vi "Spacer Position.vi"() -> ()   [LabVIEW 2020]
doc: "Este programa executa calculos para determinar o número de espaçadores e a sua respectiva posição."
uses:
  controles/SP dados de entrada.ctl
  controles/SP data.ctl
panel:
  out "Etapa":string="Término do programa"
  in  "Próximo":bool
  in  "Parar 2":bool
  out "Dados":enum32{"Dados", "Análise"}(tab)
  in  "Condutor":T1={"Pc (N/m)"=18.35, "Mod.Young (GPa)"=65.0, "Dil.Term.c (u/°C)"=20.9, "Seção trans. (mm²)"=496.0, "Tração EDS (N)"=18350.0, "Tração Lim.orig (N)"=0.0, "Tração Text (N)"=0.0} {"Tração Text (N)" min=0.0 max=1000000.0 step=0.01 format="%.2f"; "Tração Lim.orig (N)" min=0.0 max=1000000.0 step=0.01 format="%.2f"; "Pc (N/m)" min=1.0 max=100.0 step=0.01 format="%#.2g"; "Mod.Young (GPa)" min=1.0 max=500.0 step=0.001 format="%#.3f"; "Dil.Term.c (u/°C)" min=0.0 max=40.0 step=0.001 format="%#.2f"; "Seção trans. (mm²)" min=0.0 max=2000.0 step=0.001 format="%#.6f"; "Tração EDS (N)" min=1000.0 max=200000.0 step=0.01 format="%.2f"}
  in  "Suporte":T2={"Ps (N/m)"=10.0, "Mod.Young (GPa)"=112.0, "Dil.Term.c (u/°C)"=1.6, "Seção trans. (mm²)"=396.0, "Tração EDS (N)"=13250.0, "AT sup (N)"=0.0, "Flecha sup AT (m)"=0.0} {"AT sup (N)" min=0.0 max=2000.0 step=0.001 format="%#.6f"; "Tração EDS (N)" min=0.0 max=500000.0 step=0.01 format="%#.6f"; "Ps (N/m)" min=1.0 max=200.0 step=0.01; "Mod.Young (GPa)" min=1.0 max=500.0 step=0.001 format="%#.3f"; "Dil.Term.c (u/°C)" min=0.0 max=40.0 step=0.001 format="%#_3f"; "Seção trans. (mm²)" min=0.0 max=2000.0 step=0.001 format="%#.6f"}
  in  "Projeto":T3={"Temp. EDS (°C)"=25.0, "Limite orig (°C)"=60.0, "Limite est (°C)"=100.0, "N° Cabo/Fase"=4} {"N° Cabo/Fase" min=1 max=8 step=1; "Limite est (°C)" min=-50.0 max=300.0 step=0.01; "Temp. EDS (°C)" min=-50.0 max=100.0 step=0.01; "Limite orig (°C)" min=0.0 max=300.0 step=0.01}
  in  "Vão":T4={"Extensão. (m)"=700.0, "Desnível (m)"=20.0, "Ext lim subvão (m)"=20.0, "Flecha 60 (°C)"=0.0} {"Ext lim subvão (m)" min=0.0 max=500.0 step=0.01; "Flecha 60 (°C)" min=0.0 max=500.0 step=0.01; "Extensão. (m)" min=100.0 max=2000.0 step=0.01; "Desnível (m)" min=0.0 max=500.0 step=0.01}
  in  "Subaba de dados":enum32{"Espaçadores", "Subvão", "Cabo Suporte"}(tab)
  out "N Espaçadores":dbl=8.0
  out "Posição no vão (m)":dbl[](array[numeric])
  out "Tração cond. (N)":dbl=17448.399999999863
  out "Extensão c/ 55% (m)":dbl
  out "Flecha lim.calc (m)":dbl
  out "Comp Calc (m)":dbl=17448.399999999863
  out "Tração EDS (N)":dbl=83817.19488812913
  out "Tração Test (N)":dbl=83817.19488812913
  out "Flecha Test (m)":dbl
  out "Gráfico":cluster{dbl[], dbl[]}[](graph)
  in  "Gravar":bool
  # "Preenchimento de dados"
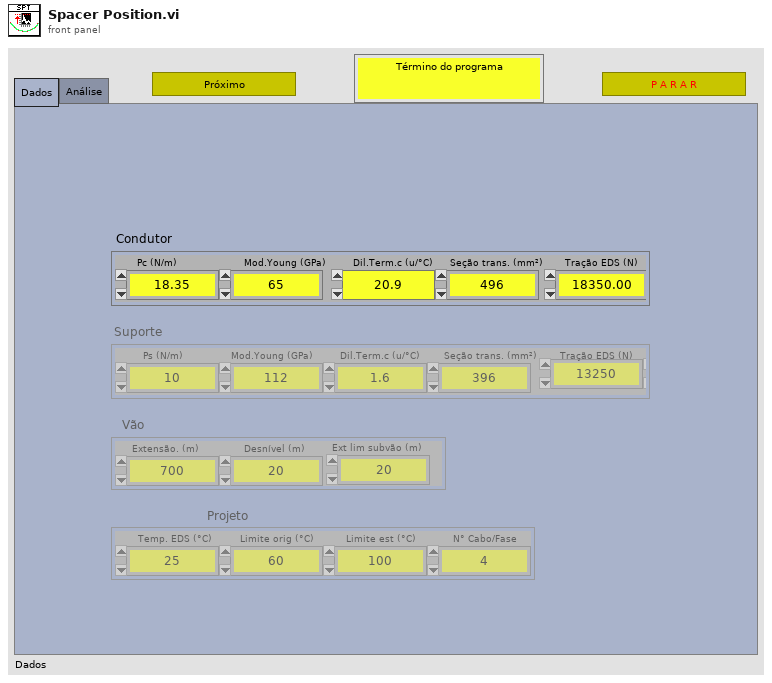
[diagram p1: front panel]
types:
  T1 = cluster{"Pc (N/m)":dbl, "Mod.Young (GPa)":dbl, "Dil.Term.c (u/°C)":dbl, "Seção trans. (mm²)":dbl, "Tração EDS (N)":dbl, "Tração Lim.orig (N)":dbl, "Tração Text (N)":dbl}
  T2 = cluster{"Ps (N/m)":dbl, "Mod.Young (GPa)":dbl, "Dil.Term.c (u/°C)":dbl, "Seção trans. (mm²)":dbl, "Tração EDS (N)":dbl, "AT sup (N)":dbl, "Flecha sup AT (m)":dbl}
  T3 = cluster{"Temp. EDS (°C)":dbl, "Limite orig (°C)":dbl, "Limite est (°C)":dbl, "N° Cabo/Fase":u32}
  T4 = cluster{"Extensão. (m)":dbl, "Desnível (m)":dbl, "Ext lim subvão (m)":dbl, "Flecha 60 (°C)":dbl}
  T5 = typedef "SP data.ctl" = cluster{"Condutor":cluster{"Pc (N/m)":dbl, "Mod.Young (N/m²)":dbl, "Dil.Term.c (m/°C)":dbl, "Área  (m²)":dbl, "Tração EDS (N)":dbl, "Tração Torig(N)":dbl, "Tração Talta (N)":dbl}, "Suporte":cluster{"Ps (N/m)":dbl, "Es (N/m²)":dbl, "DTc (1/°C)":dbl, "Área sup (m²)":dbl, "Tração EDS sup (N)":dbl, "Tração AT sup (N)":dbl, "Flecha sup AT (m)":dbl}, "Projeto":cluster{"Temp. EDS (°C)":dbl, "Lim.original (°C)":dbl, "Lim.extend. (°C)":dbl, "N. cabo/fase":dbl}, "Vetor de dados":cluster{"Coor.X.esp":dbl[], "Coor.Y.Esp.":dbl[], "Sub.vao X":dbl[], "Sub.vao Y":dbl[], "CoordY.sup":dbl[], "CoordX.sup":dbl[]}, "Subvão":cluster{"N. Esp.":dbl, "F.lim (m)":dbl, "Ext.calc":dbl, "Ext.definido":dbl, "Comp.cabo":dbl, "Ext.55%":dbl, "Tração sub\nAT (N)":dbl, "Ext.sel.":dbl, "Flecha lim.\ncalc (m)":dbl}, "Vão":cluster{"Extensão (m)":dbl, "Desnivel (m)":dbl, "Ext.Lim sub (m)":dbl, "Flecha à 60 °C":dbl}}
  T6 = typedef "SP dados de entrada.ctl" = enum16{"Iniciar", "Aguardar", "Condutor", "Suporte", "Vão", "Projeto", "Atualizar UI", "Mensagem", "Calcular", "Análise dos dados", "Fim"}
  T7 = enum8{"Enabled", "Disabled", "Disabled and Grayed Out"}
  T8 = cluster{"CoordX.sup":dbl[], "CoordY.sup":dbl[]}[]
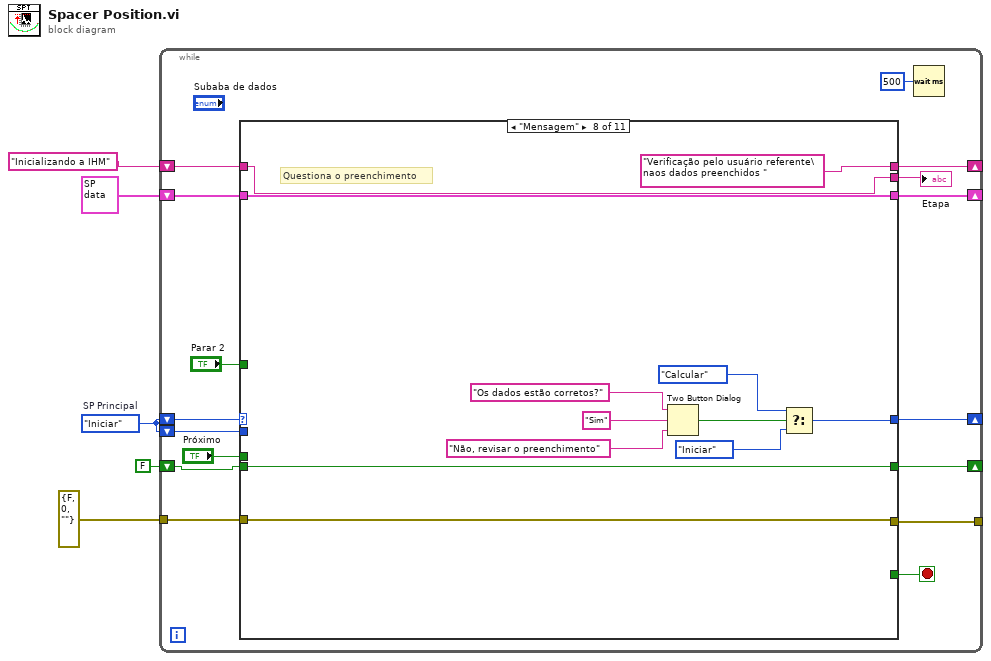
[diagram p0: block diagram]
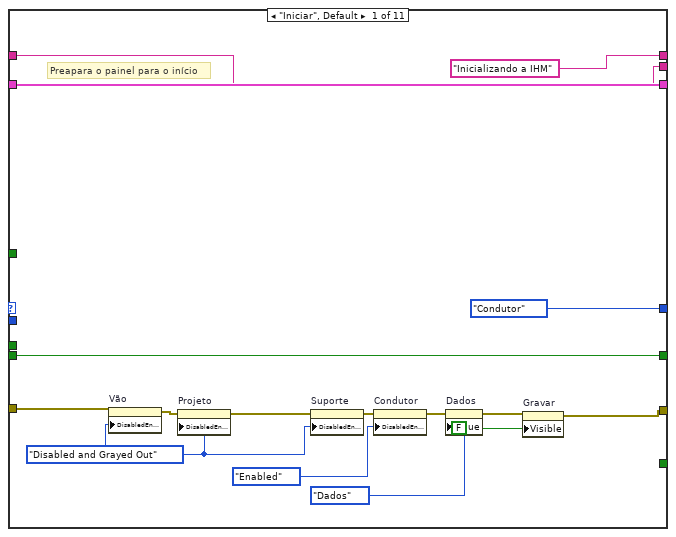
[diagram p2: hidden frame]
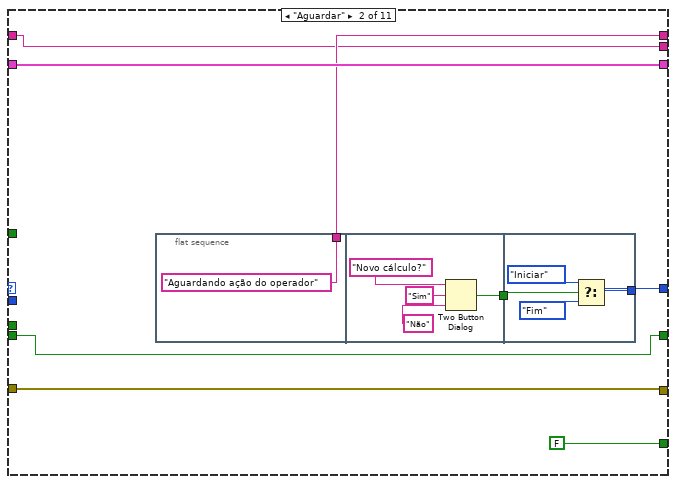
[diagram p3: hidden frame]
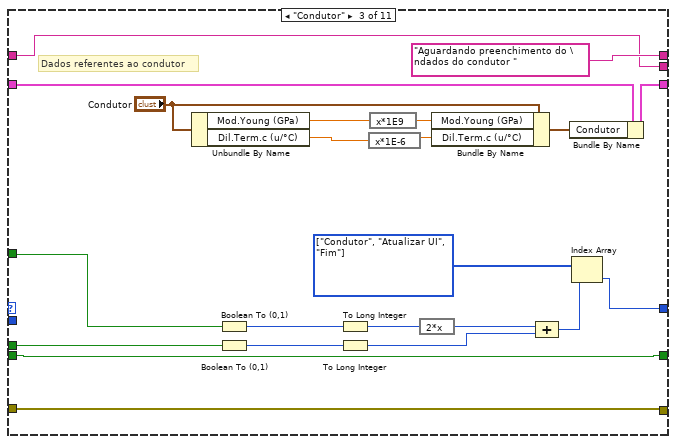
[diagram p4: hidden frame]
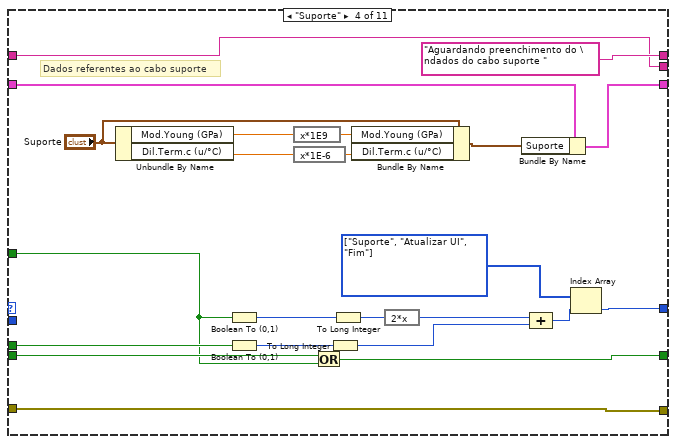
[diagram p5: hidden frame]
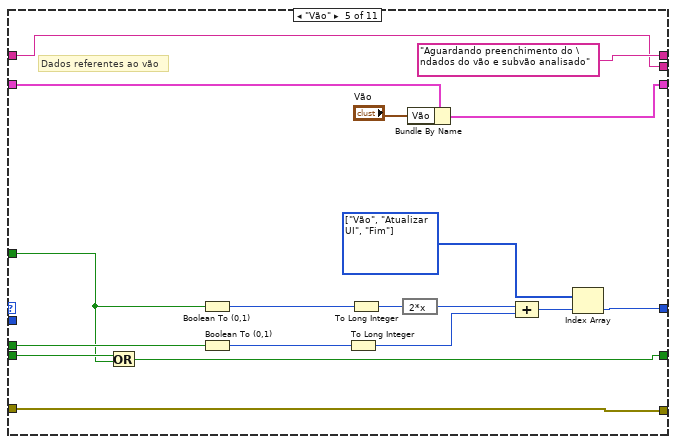
[diagram p6: hidden frame]
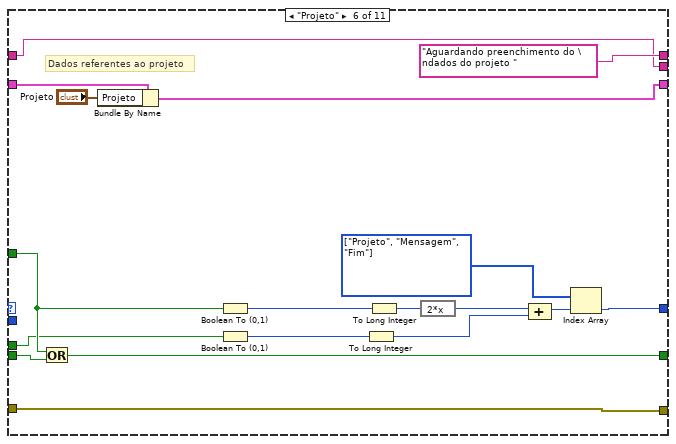
[diagram p7: hidden frame]
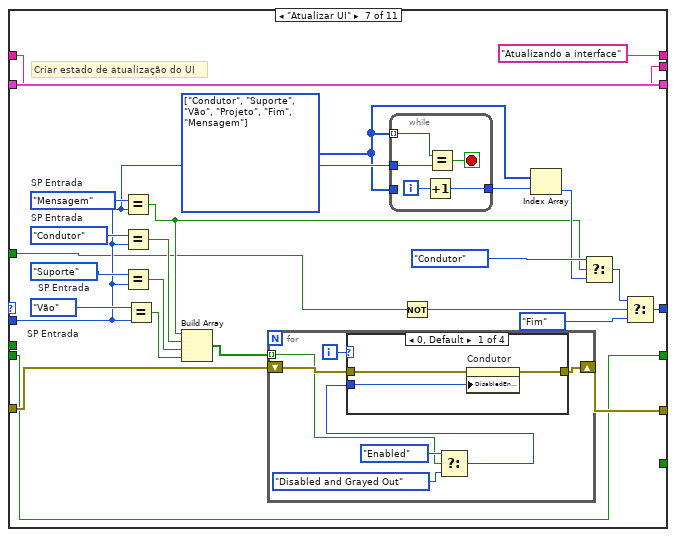
[diagram p8: hidden frame]
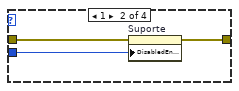
[diagram p9: hidden frame]
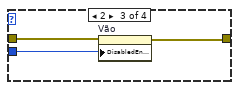
[diagram p10: hidden frame]
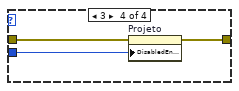
[diagram p11: hidden frame]
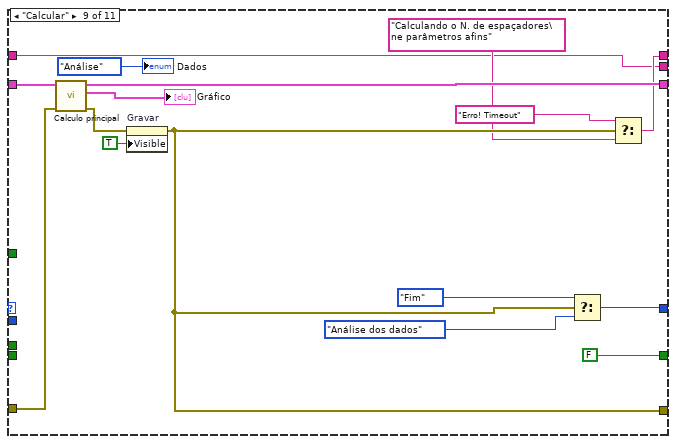
[diagram p12: hidden frame]
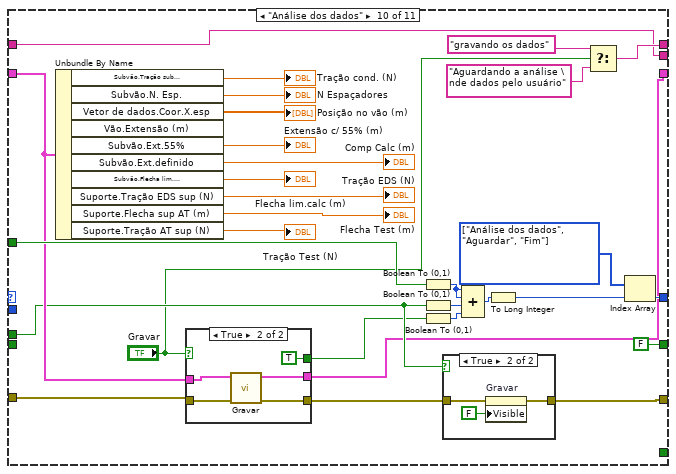
[diagram p13: hidden frame]
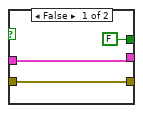
[diagram p14: hidden frame]
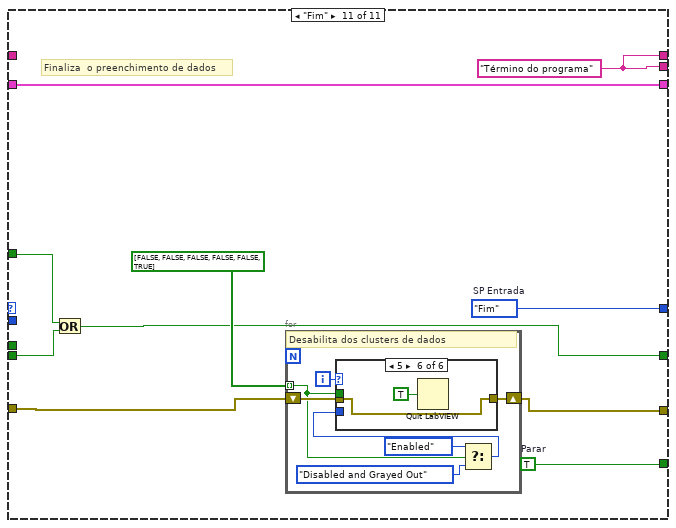
[diagram p16: hidden frame]
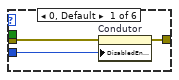
[diagram p17: hidden frame]
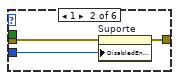
[diagram p18: hidden frame]
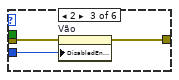
[diagram p19: hidden frame]
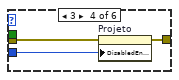
[diagram p20: hidden frame]
diagram:
  w3 = SP_dados_de_entrada."Iniciar"  # SP Principal
  n1 = while {
    shift-right: [w20] -> _
    shift-left: w3 -> [w21]
    shift-right: [w17] -> _
    shift-left: T5 {"Condutor"={"Pc (N/m)"=0.0, "Mod.Young (N/m²)"=0.0, "Dil.Term.c (m/°C)"=0.0, "Área  (m²)"=0.0, "Tração EDS (N)"=0.0, "Tração Torig(N)"=0.0, "Tração Talta (N)"=0.0}, "Suporte"={"Ps (N/m)"=0.0, "Es (N/m²)"=0.0, "DTc (1/°C)"=0.0, "Área sup (m²)"=0.0, "Tração EDS sup (N)"=0.0, "Tração AT sup (N)"=0.0, "Flecha sup AT (m)"=0.0}, "Projeto"={"Temp. EDS (°C)"=0.0, "Lim.original (°C)"=0.0, "Lim.extend. (°C)"=0.0, "N. cabo/fase"=1.0}, "Vetor de dados"={"Coor.X.esp"=[], "Coor.Y.Esp."=[], "Sub.vao X"=[], "Sub.vao Y"=[], "CoordY.sup"=[], "CoordX.sup"=[]}, "Subvão"={"N. Esp."=0.0, "F.lim (m)"=0.0, "Ext.calc"=0.0, "Ext.definido"=0.0, "Comp.cabo"=0.0, "Ext.55%"=0.0, "Tração sub\nAT (N)"=0.0, "Ext.sel."=0.0, "Flecha lim.\ncalc (m)"=0.0}, "Vão"={"Extensão (m)"=0.0, "Desnivel (m)"=0.0, "Ext.Lim sub (m)"=0.0, "Flecha à 60 °C"=0.0}} ("SP Dados In") -> [w18]
    shift-left: w3 -> [w15]
    tunnel: errorcluster {"status"=FALSE, "code"=0, "source"=""} ("error in") -> [w14]
    tunnel: [w9] -> _
    shift-right: [w12] -> _
    shift-left: FALSE ("T button?") -> [w11]
    shift-right: [w8] -> _
    shift-left: "Inicializando a IHM" ("Etapa") -> [w6]
    stop <- w19 stop-if-true
    n2 = case shown="\"Mensagem\"" w21 {
      tunnel: [SP_dados_de_entrada."Condutor" ("SP Entrada") w39 w73 w98 w116 w134 w149 w192 w201 w230 w264] -> w20
      tunnel: [_ FALSE ("Parar") _ _ _ _ _ _ _ _ w263] -> w19
      tunnel: [w37 w45 w74 w77 w114 w119 w157 w186 w207 w221 w262] -> w17
      tunnel: w18 -> [w37 w45 w75 w79 w115 w133 w157 w186 w211 w225 w262]
      tunnel: w15 -> [_ _ _ _ _ _ w142 _ _ _ _]
      tunnel: w14 -> [w23 w43 w72 w97 w113 w131 w153 w195 w210 w226 w261]
      tunnel: [w28 w43 w72 w97 w113 w131 w152 w195 w206 w222 w260] -> w9
      tunnel: "Próximo" -> [_ _ w70 w95 w103 w120 _ _ _ w224 _]
      tunnel: [w33 w44 w69 w93 w111 w130 w140 w188 FALSE ("T button?") FALSE ("T button?") w258] -> w12
      tunnel: w11 -> [w33 w44 w69 w94 w112 w122 w140 w188 _ _ w257]
      tunnel: "Parar 2" -> [_ _ w63 w88 w102 w121 w139 _ _ w228 w256]
      tunnel: ["Inicializando a IHM" ("Etapa") w41 "Aguardando preenchimento do \ndados do condutor " ("Etapa") "Aguardando preenchimento do \ndados do cabo suporte " ("Etapa") "Aguardando preenchimento do \ndados do vão e subvão analisado" ("Etapa") "Aguardando preenchimento do \ndados do projeto " ("Etapa") "Atualizando a interface" ("Etapa") "Verificação pelo usuário referente\naos dados preenchidos " ("Etapa") w199 w217 w255] -> w8
      tunnel: [w25 w38 w61 w85 w101 w118 w136 w185 w197 w213 w255] -> w7
      tunnel: w6 -> [w25 w38 w61 w85 w101 w118 w136 w185 w197 w213 _]
      frame "Iniciar", Default {
        w22 = T7."Disabled and Grayed Out" ("Disabled")
        # "Preapara o painel para o início"
        n3 = property on="Vão" class="Clust (strict)"(error in=w23, "DisabledEnum"=w22) -> (error out=w24:errorcluster)  [unwired: 1 in, 1 out]
        n4 = property on="Projeto" class="Clust (strict)"(error in=w24, "DisabledEnum"=w22) -> (error out=w36:errorcluster)  [unwired: 1 in, 1 out]
        n5 = property on="Suporte" class="Clust (strict)"(error in=w36, "DisabledEnum"=w22) -> (error out=w35:errorcluster)  [unwired: 1 in, 1 out]
        n6 = property on="Condutor" class="Clust (strict)"(error in=w35, "DisabledEnum"=T7."Enabled" ("Disabled")) -> (error out=w32:errorcluster)  [unwired: 1 in, 1 out]
        n7 = property on="Dados" class="TabCtl (strict)"(error in=w32, "Value"=enum32{"Dados", "Análise"}."Dados" ("Dados")) -> (error out=w29:errorcluster)  [unwired: 1 in, 1 out]
        n8 = property on="Gravar" class="Bool"(error in=w29, "Visible"=FALSE) -> (error out=w28:errorcluster)  [unwired: 1 in, 1 out]
      }
      frame "Aguardar" {
        n9 = flat-sequence {
          tunnel: ["Aguardando ação do operador" ("Etapa")] -> w41
          tunnel: [w47] -> w40
          tunnel: w40 -> [w53]
          tunnel: [w51] -> w39
          frame #0 {
          }
          frame #1 {
            n10 = Two Button Dialog(message="Novo cálculo?" ("T button name (\"OK\")"), 1:"Não" ("F button name (\"Cancel\")"), 2:"Sim" ("message")) -> (T button?=w47:bool)
          }
          frame #2 {
            n11 = Select(t=SP_dados_de_entrada."Iniciar" ("SP Entrada"), s=w53, f=SP_dados_de_entrada."Fim" ("SP Entrada")) -> (s? t:f=w51:T6)
          }
        }
      }
      frame "Condutor" {
        w76 = T6[] [enum."Condutor", enum."Atualizar UI", enum."Fim"] items=["Iniciar", "Aguardar", "Condutor", "Suporte", "Vão", "Projeto", "Atualizar UI", "Mensagem", "Calcular", "Análise dos dados", "Fim"]
        # "Dados referentes ao condutor"
        n12 = Unbundle By Name("Condutor") -> ("Mod.Young (GPa)"=w59:dbl, "Dil.Term.c (u/°C)"=w56:dbl)
        n13 = Boolean To (0,1)(Boolean=w63) -> (0, 1=w65:i16)
        n14 = Boolean To (0,1)(Boolean=w70) -> (0, 1=w71:i16)
        n15 = To Long Integer(number=w65) -> (32bit integer=w64:i32)
        n16 = To Long Integer(number=w71) -> (32bit integer=w67:i32)
        n17 = expression code="x*1E-6"(w56) -> (w55:dbl)
        n18 = expression code="x*1E9"(w59) -> (w58:dbl)
        n19 = expression code="2*x"(w64) -> (w62:i32)
        n20 = Bundle By Name(cluster="Condutor", "Mod.Young (GPa)"=w58, "Dil.Term.c (u/°C)"=w55) -> (w57:T1)
        n21 = Compound Arithmetic op=ADD(w62, w67) -> (w66:i32)
        n22 = Bundle By Name(cluster=w75, "Condutor"=w57) -> (w74:T5)
        n23 = Index Array(array=w76, index=w66) -> (element=w73:T6)
      }
      frame "Suporte" {
        w99 = T6[] [enum."Suporte", enum."Atualizar UI", enum."Fim"] items=["Iniciar", "Aguardar", "Condutor", "Suporte", "Vão", "Projeto", "Atualizar UI", "Mensagem", "Calcular", "Análise dos dados", "Fim"]
        # "Dados referentes ao cabo suporte"
        n24 = Unbundle By Name("Suporte") -> ("Mod.Young (GPa)"=w84:dbl, "Dil.Term.c (u/°C)"=w82:dbl)
        n25 = Boolean To (0,1)(Boolean=w88) -> (0, 1=w91:i16)
        n26 = Boolean To (0,1)(Boolean=w95) -> (0, 1=w96:i16)
        n27 = expression code="x*1E9"(w84) -> (w83:dbl)
        n28 = expression code="x*1E-6"(w82) -> (w81:dbl)
        n29 = Or(x=w94, y=w88) -> (x .or. y?=w93:bool)
        n30 = To Long Integer(number=w96) -> (32bit integer=w87:i32)
        n31 = To Long Integer(number=w91) -> (32bit integer=w90:i32)
        n32 = Bundle By Name(cluster="Suporte", "Mod.Young (GPa)"=w83, "Dil.Term.c (u/°C)"=w81) -> (w78:T2)
        n33 = expression code="2*x"(w90) -> (w89:i32)
        n34 = Bundle By Name(cluster=w79, "Suporte"=w78) -> (w77:T5)
        n35 = Compound Arithmetic op=ADD(w89, w87) -> (w86:i32)
        n36 = Index Array(array=w99, index=w86) -> (element=w98:T6)
      }
      frame "Vão" {
        w117 = T6[] [enum."Vão", enum."Atualizar UI", enum."Fim"] items=["Iniciar", "Aguardar", "Condutor", "Suporte", "Vão", "Projeto", "Atualizar UI", "Mensagem", "Calcular", "Análise dos dados", "Fim"]
        # "Dados referentes ao vão"
        n37 = Or(x=w112, y=w102) -> (x .or. y?=w111:bool)
        n38 = Boolean To (0,1)(Boolean=w102) -> (0, 1=w108:i16)
        n39 = Boolean To (0,1)(Boolean=w103) -> (0, 1=w109:i16)
        n40 = To Long Integer(number=w109) -> (32bit integer=w105:i32)
        n41 = To Long Integer(number=w108) -> (32bit integer=w107:i32)
        n42 = expression code="2*x"(w107) -> (w106:i32)
        n43 = Bundle By Name(cluster=w115, "Vão"="Vão") -> (w114:T5)
        n44 = Compound Arithmetic op=ADD(w106, w105) -> (w104:i32)
        n45 = Index Array(array=w117, index=w104) -> (element=w116:T6)
      }
      frame "Projeto" {
        w135 = T6[] [enum."Projeto", enum."Mensagem", enum."Fim"] items=["Iniciar", "Aguardar", "Condutor", "Suporte", "Vão", "Projeto", "Atualizar UI", "Mensagem", "Calcular", "Análise dos dados", "Fim"]
        # "Dados referentes ao projeto"
        n46 = Or(x=w121, y=w122) -> (x .or. y?=w130:bool)
        n47 = Bundle By Name(cluster=w133, "Projeto"="Projeto") -> (w119:T5)
        n48 = Boolean To (0,1)(Boolean=w121) -> (0, 1=w127:i16)
        n49 = Boolean To (0,1)(Boolean=w120) -> (0, 1=w128:i16)
        n50 = To Long Integer(number=w128) -> (32bit integer=w124:i32)
        n51 = To Long Integer(number=w127) -> (32bit integer=w126:i32)
        n52 = expression code="2*x"(w126) -> (w125:i32)
        n53 = Compound Arithmetic op=ADD(w125, w124) -> (w123:i32)
        n54 = Index Array(array=w135, index=w123) -> (element=w134:T6)
      }
      frame "Atualizar UI" {
        w147 = SP_dados_de_entrada."Mensagem"  # SP Entrada
        w138 = T6[] [enum."Condutor", enum."Suporte", enum."Vão", enum."Projeto", enum."Fim", enum."Mensagem"] items=["Iniciar", "Aguardar", "Condutor", "Suporte", "Vão", "Projeto", "Atualizar UI", "Mensagem", "Calcular", "Análise dos dados", "Fim"]
        w158 = SP_dados_de_entrada."Vão"  # SP Entrada
        w159 = SP_dados_de_entrada."Suporte"  # SP Entrada
        w160 = SP_dados_de_entrada."Condutor"  # SP Entrada
        # "Criar estado de atualização do UI"
        n55 = Equal?(x=w147, y=w142) -> (x = y?=w141:bool)
        n56 = Equal?(x=w160, y=w142) -> (x = y?=w156:bool)
        n57 = Equal?(x=w159, y=w142) -> (x = y?=w155:bool)
        n58 = Equal?(x=w158, y=w142) -> (x = y?=w148:bool)
        n59 = Build Array(w141, w156, w155, w148) -> (w154:bool[])
        n60 = for {
          shift-right: [w166] -> w152
          shift-left: w153 -> [w165]
          tunnel: w154 -> [w161] mode=indexing
          i -> [w167]
          n61 = Select(t=T7."Enabled" ("Disabled"), s=w161, f=T7."Disabled and Grayed Out" ("Disabled")) -> (s? t:f=w162:T7)
          n62 = case shown="0, Default" w167 {
            tunnel: [w170 w173 w175 w179] -> w166
            tunnel: w165 -> [w168 w172 w174 w178]
            tunnel: w162 -> [w169 w171 w176 w177]
            frame 0, Default {
              n63 = property on="Condutor" class="Clust (strict)"(error in=w168, "DisabledEnum"=w169) -> (error out=w170:errorcluster)  [unwired: 1 in, 1 out]
            }
            frame 1 {
              n64 = property on="Suporte" class="Clust (strict)"(error in=w172, "DisabledEnum"=w171) -> (error out=w173:errorcluster)  [unwired: 1 in, 1 out]
            }
            frame 2 {
              n65 = property on="Vão" class="Clust (strict)"(error in=w174, "DisabledEnum"=w176) -> (error out=w175:errorcluster)  [unwired: 1 in, 1 out]
            }
            frame 3 {
              n66 = property on="Projeto" class="Clust (strict)"(error in=w178, "DisabledEnum"=w177) -> (error out=w179:errorcluster)  [unwired: 1 in, 1 out]
            }
          }
        }
        n67 = while {
          tunnel: w138 -> [w180] mode=indexing
          tunnel: w138 -> [_]
          tunnel: [w182] -> w146
          tunnel: w142 -> [w181]
          i -> [w183]
          stop <- w184 stop-if-true
          n68 = Increment(x=w183) -> (x+1=w182:i32)
          n69 = Equal?(x=w180, y=w181) -> (x = y?=w184:bool)
        }
        n70 = Not(x=w139) -> (.not. x?=w151:bool)
        n71 = Index Array(array=w138, index=w146) -> (element=w144:T6)
        n72 = Select(t=SP_dados_de_entrada."Condutor" ("f"), s=w141, f=w144) -> (s? t:f=w143:T6)
        n73 = Select(t=w143, s=w151, f=SP_dados_de_entrada."Fim") -> (s? t:f=w149:T6)
      }
      frame "Mensagem" {
        # "Questiona o preenchimento"
        n74 = Two Button Dialog(message="Os dados estão corretos?" ("T button name (\"OK\")"), 1:"Não, revisar o preenchimento" ("F button name (\"Cancel\")"), 2:"Sim" ("message")) -> (T button?=w189:bool)
        n75 = Select(t=SP_dados_de_entrada."Calcular" ("SP Entrada"), s=w189, f=SP_dados_de_entrada."Iniciar" ("SP Entrada")) -> (s? t:f=w192:T6)
      }
      frame "Calcular" {
        n76 = call "Calculo principal.vi"("error in"=w210, "Dados SP"=w211) -> ("error out"=w208:errorcluster, "Gráfico"=→"Gráfico":T8, "Dados SP Out"=w207:T5)  [unwired: 7 in]
        n77 = property on="Gravar" class="Bool"(error in=w208, "Visible"=TRUE) -> (error out=w206:errorcluster)  [unwired: 1 in, 1 out]
        n78 = Select(t=SP_dados_de_entrada."Fim", s=w206, f=SP_dados_de_entrada."Análise dos dados" ("SP Entrada")) -> (s? t:f=w201:T6)
        n79 = Select(t="Erro! Timeout", s=w206, f="Calculando o N. de espaçadores\ne parâmetros afins" ("Etapa")) -> (s? t:f=w199:string)
        "Dados" <- enum32{"Dados", "Análise"}."Análise" ("Dados")
      }
      frame "Análise dos dados" {
        w233 = T6[] [enum."Análise dos dados", enum."Aguardar", enum."Fim"] items=["Iniciar", "Aguardar", "Condutor", "Suporte", "Vão", "Projeto", "Atualizar UI", "Mensagem", "Calcular", "Análise dos dados", "Fim"]
        n80 = Unbundle By Name(w225) -> ("Subvão.Tração sub\nAT (N)"=→"Tração cond. (N)":dbl, "Subvão.N. Esp."=→"N Espaçadores":dbl, "Vetor de dados.Coor.X.esp"=→"Posição no vão (m)":dbl[], "Subvão.Ext.55%"=→"Extensão c/ 55% (m)":dbl, "Subvão.Ext.definido"=→"Comp Calc (m)":dbl, "Subvão.Flecha lim.\ncalc (m)"=→"Flecha lim.calc (m)":dbl, "Suporte.Tração EDS sup (N)"=→"Tração EDS (N)":dbl, "Suporte.Flecha sup AT (m)"=→"Flecha Test (m)":dbl, "Suporte.Tração AT sup (N)"=→"Tração Test (N)":dbl)  [unwired: 1 out]
        n81 = case shown="True" "Gravar" {
          tunnel: w225 -> [w245 w250]
          tunnel: [w245 w249] -> w221
          tunnel: w226 -> [w244 w248]
          tunnel: [w244 w247] -> w223
          tunnel: [FALSE ("Boolean") TRUE ("Boolean")] -> w218
          frame False {
          }
          frame True {
            n82 = call "Gravar.vi"("error in (no error)"=w248, "SP Dados In"=w250) -> ("error out"=w247:errorcluster, "SP Dados Out"=w249:T5)  [unwired: 8 in]
          }
        }
        n83 = Boolean To (0,1)(Boolean=w228) -> (0, 1=w227:i16)
        n84 = Boolean To (0,1)(Boolean=w224) -> (0, 1=w232:i16)
        n85 = Boolean To (0,1)(Boolean=w218) -> (0, 1=w219:i16)
        n86 = case shown="True" w224 {
          tunnel: w223 -> [w251 w254]
          tunnel: [w251 w253] -> w222
          frame False {
          }
          frame True {
            n87 = property on="Gravar" class="Bool"(error in=w254, "Visible"=FALSE) -> (error out=w253:errorcluster)  [unwired: 1 in, 1 out]
          }
        }
        n88 = Compound Arithmetic op=ADD(w227, w227, w232, w219) -> (w229:i16)
        n89 = To Long Integer(number=w229) -> (32bit integer=w231:i32)
        n90 = Select(t="gravando os dados" ("Etapa"), s="Gravar", f="Aguardando a análise \nde dados pelo usuário" ("Etapa")) -> (s? t:f=w217:string)
        n91 = Index Array(array=w233, index=w231) -> (element=w230:T6)
      }
      frame "Fim" {
        w255 = "Término do programa" ("Etapa")
        w263 = TRUE  # Parar
        w264 = SP_dados_de_entrada."Fim"  # SP Entrada
        # "Finaliza  o preenchimento de dados"
        n92 = Or(x=w256, y=w257) -> (x .or. y?=w258:bool)
        n93 = for {
          shift-right: [w270] -> w260
          shift-left: w261 -> [w269]
          tunnel: bool[] [FALSE, FALSE, FALSE, FALSE, FALSE, TRUE] -> [w265] mode=indexing
          i -> [w271]
          # "Desabilita dos clusters de dados"
          n94 = Select(t=T7."Enabled" ("Disabled"), s=w265, f=T7."Disabled and Grayed Out" ("Disabled")) -> (s? t:f=w266:T7)
          n95 = case shown="5" w271 {
            tunnel: [w274 w277 w280 w283 w286 w288] -> w270
            tunnel: w269 -> [w272 w276 w278 w282 w285 w288]
            tunnel: w266 -> [w273 w275 w279 w281 _ _]
            tunnel: w265 -> [_ _ _ _ _ _]
            frame 0, Default {
              n96 = property on="Condutor" class="Clust (strict)"(error in=w272, "DisabledEnum"=w273) -> (error out=w274:errorcluster)  [unwired: 1 in, 1 out]
            }
            frame 1 {
              n97 = property on="Suporte" class="Clust (strict)"(error in=w276, "DisabledEnum"=w275) -> (error out=w277:errorcluster)  [unwired: 1 in, 1 out]
            }
            frame 2 {
              n98 = property on="Vão" class="Clust (strict)"(error in=w278, "DisabledEnum"=w279) -> (error out=w280:errorcluster)  [unwired: 1 in, 1 out]
            }
            frame 3 {
              n99 = property on="Projeto" class="Clust (strict)"(error in=w282, "DisabledEnum"=w281) -> (error out=w283:errorcluster)  [unwired: 1 in, 1 out]
            }
            frame 4 {
              n100 = property on="Gravar" class="Bool"(error in=w285, "Visible"=FALSE) -> (error out=w286:errorcluster)  [unwired: 1 in, 1 out]
            }
            frame 5 {
              n101 = Quit LabVIEW(quit? (T)=TRUE) -> ()
            }
          }
        }
      }
    }
    "Etapa" <- w7
    n102 = Wait (ms)(milliseconds to wait=u32 500) -> ()  [unwired: 1 out]
  }
